vi "Convolucion.vi"() -> ()   [LabVIEW 2017]
panel:
  in  "Vertical Fill Slide":dbl(slide) scale=-4.0..4.0
  out "XY Graph 3":cluster{dbl[], dbl[]}[](graph)
  out "XY Graph 2":cluster{dbl[], dbl[]}(graph)
  out "XY Graph":cluster{dbl[], dbl[]}(graph)
  in  "df":dbl
  in  "to":dbl
  in  "tf":dbl
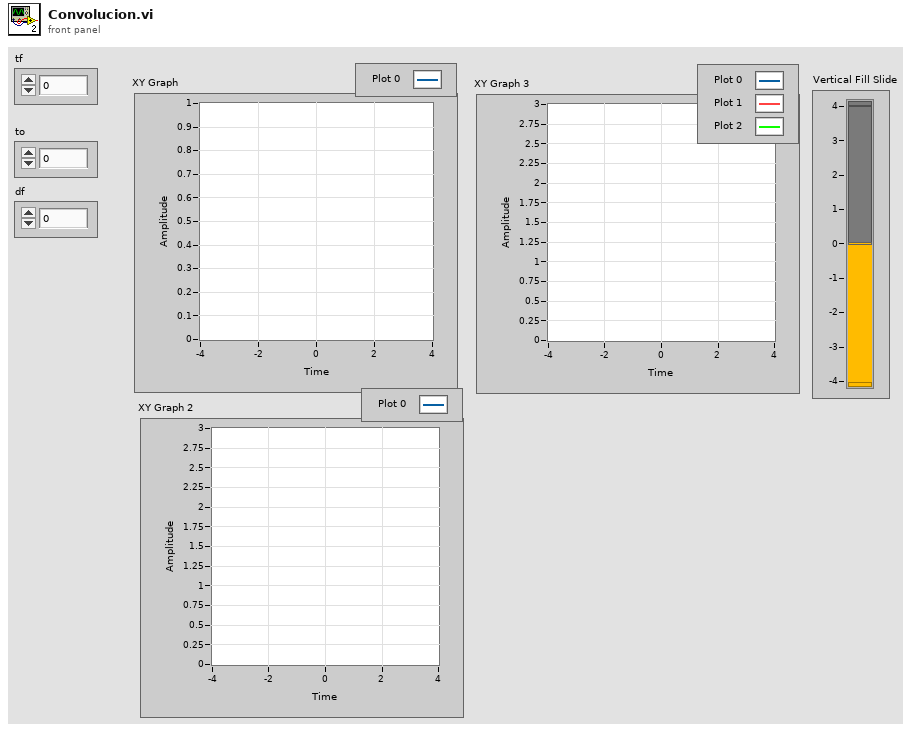
[diagram p1: front panel]
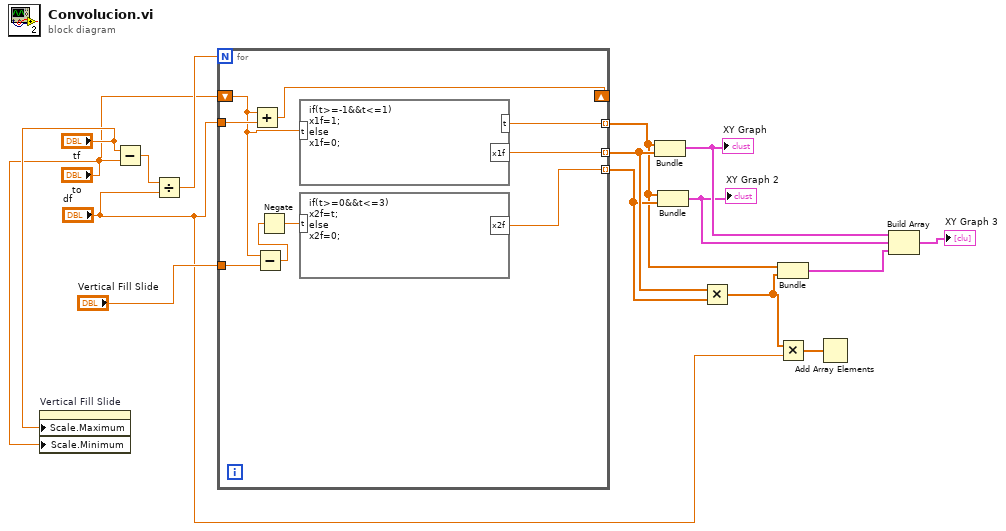
[diagram p0: block diagram]
diagram:
  n1 = property on="Vertical Fill Slide" class="Slide (strict)"("Scale.Maximum"="tf", "Scale.Minimum"="to") -> ()  [unwired: 2 in, 2 out]
  n2 = Subtract(x="tf", y="to") -> (x-y=w15:dbl)
  n3 = Divide(x=w15, y="df") -> (x/y=w14:dbl)
  n4 = for {
    N: w14 -> [_]
    shift-right: [w24] -> _
    shift-left: "to" -> [w18]
    tunnel: "df" -> [w23]
    tunnel: [w22] -> w9 mode=indexing
    tunnel: [w21] -> w6 mode=indexing
    tunnel: [w20] -> w8 mode=indexing
    tunnel: "Vertical Fill Slide" -> [w19]
    n5 = Add(x=w18, y=w23) -> (x+y=w24:dbl)
    n6 = Subtract(x=w18, y=w19) -> (x-y=w17:dbl)
    n7 = Negate(x=w17) -> (-x=w16:dbl)
    n8 = formula code="if(t>=-1&&t<=1)\nx1f=1;\nelse\nx1f=0;"("t"=w18) -> ("x1f"=w22:dbl, "t"=w21:dbl)
    n9 = formula code="if(t>=0&&t<=3)\nx2f=t;\nelse\nx2f=0;"("t"=w16) -> ("x2f"=w20:dbl)
  }
  n10 = Bundle(w6, w9) -> (w13:cluster{dbl[], dbl[]})  [unwired: 1 in]
  "XY Graph" <- w13
  n11 = Bundle(w6, w8) -> (w12:cluster{dbl[], dbl[]})  [unwired: 1 in]
  "XY Graph 2" <- w12
  n12 = Multiply(x=w9, y=w8) -> (x*y=w7:dbl[])
  n13 = Bundle(w6, w7) -> (w5:cluster{dbl[], dbl[]})  [unwired: 1 in]
  n14 = Multiply(x=w7, y="df") -> (x*y=w3:dbl[])
  n15 = Add Array Elements(numeric array=w3) -> ()  [unwired: 1 out]
  n16 = Build Array(w13, w12, w5) -> (→"XY Graph 3":cluster{dbl[], dbl[]}[])
